vi "RQST Lookup Table Initialize.vi"(8 "error in (no error)":errorcluster) -> (0 "error out":errorcluster {"code" min=0 max=0}, 3 "reference out":T1)   [LabVIEW 2013, in "J1939.lvlib"]
uses:
  J1939.lvlib
  RQST Lookup Table Reference.ctl
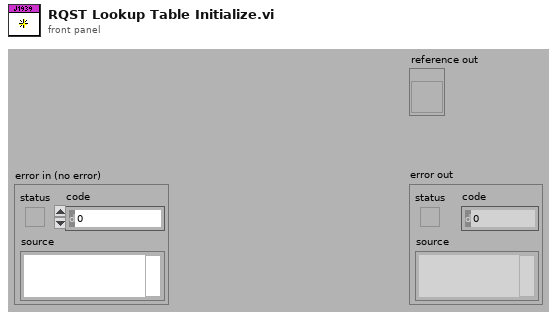
[diagram p1: front panel]
types:
  T1 = typedef "J1939.lvlib/RQST Lookup Table Reference.ctl" = refnum<vi>
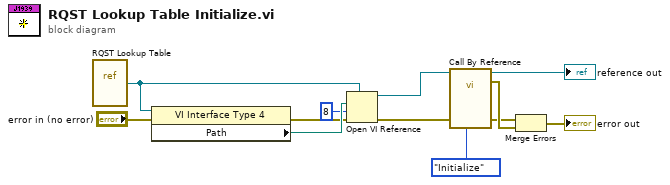
[diagram p0: block diagram]
diagram:
  n1 = vi-ref "RQST Lookup Table.vi"() -> (w12:refnum<vi>)
  n2 = property class="VI Interface Type 4"(reference=w12, error in="error in (no error)") -> (error out=w9:errorcluster, "Path"=w11:path)  [unwired: 1 out]
  n3 = Open VI Reference(type specifier VI Refnum (for type only)=w12, vi path=w11, options=8, error in (no error)=w9) -> (vi reference=w2:refnum<vi>, error out=w5:errorcluster)  [unwired: 2 in]
  n4 = call-by-ref "?"(reference=w2, "Action"=enum16{"Initialize", "Add", "Get", "Remove"}."Initialize", "error in (no error)"=w5) -> (reference out=→"reference out":refnum<vi>, error out=w8:errorcluster, 0:"error out"=w4:errorcluster)  [unwired: 8 in, 2 out]
  n5 = Merge Errors(w4, w8) -> (→"error out":errorcluster)
